vi "SecondaryJoystickButtonMapping.vi"(0 "Secondary joystick buttons":bool[](array[boolean])) -> (4 "SecondaryJoystickButtons":T1, 14 "Secondary joystick buttons indicator":bool[](array[boolean]))   [LabVIEW 2018]
uses:
  SecondaryJoystickButtons.ctl
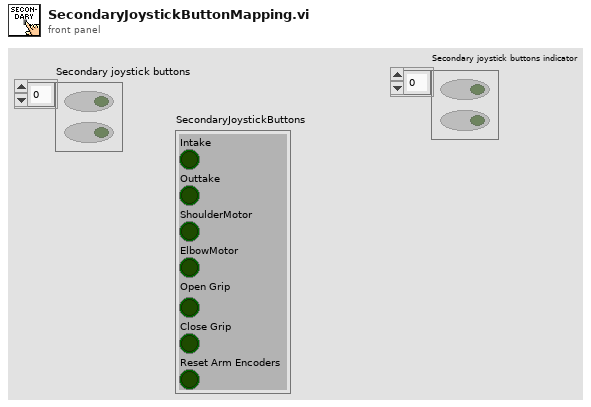
[diagram p1: front panel]
types:
  T1 = typedef "SecondaryJoystickButtons.ctl" = cluster{"Intake":bool, "Outtake":bool, "ShoulderMotor":bool, "ElbowMotor":bool, "Open Grip":bool, "Close Grip":bool, "Reset Arm Encoders":bool}
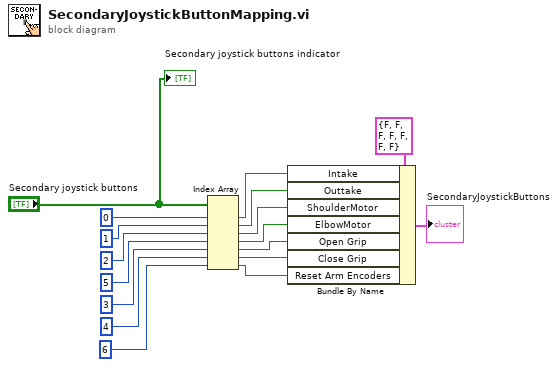
[diagram p0: block diagram]
diagram:
  n1 = Index Array(array="Secondary joystick buttons", index #1=0 ("index"), index #2=1 ("index"), index #3=2 ("index"), index #4=5 ("index"), index #5=3 ("index"), index #6=4 ("index"), index #7=6 ("index")) -> (element #1=w8:bool, element #2=w7:bool, element #3=w6:bool, element #4=w5:bool, element #5=w4:bool, element #6=w3:bool, element #7=w2:bool)
  n2 = Bundle By Name(cluster=T1 {"Intake"=FALSE, "Outtake"=FALSE, "ShoulderMotor"=FALSE, "ElbowMotor"=FALSE, "Open Grip"=FALSE, "Close Grip"=FALSE, "Reset Arm Encoders"=FALSE} ("SecondaryJoystickButtons"), "Intake"=w8, "Outtake"=w7, "ShoulderMotor"=w6, "ElbowMotor"=w5, "Open Grip"=w4, "Close Grip"=w3, "Reset Arm Encoders"=w2) -> (→"SecondaryJoystickButtons":T1)
  "Secondary joystick buttons indicator" <- "Secondary joystick buttons"
